vi "set shutdown.vi"(7 "system status in":T1={"system state"=enum."Empty & Closed", "fuel level"=0.0, "LOX level"=0.0, "system warnings"={"oxidizer overpress"=FALSE, "oxidizer leak"=FALSE, "fuel overpress"=FALSE, "fuel leak"=FALSE}, "valves"={"fuel load"=FALSE, "fuel return"=FALSE, "fuel comb"=FALSE, "fuel dump"=FALSE, "LOX load"=FALSE, "LOX return"=FALSE, "LOX comb"=FALSE, "LOX dump"=FALSE}, "ignition"=FALSE}) -> (8 "system status out":T1={"system state"=enum."Empty & Closed", "fuel level"=0.0, "LOX level"=0.0, "system warnings"={"oxidizer overpress"=FALSE, "oxidizer leak"=FALSE, "fuel overpress"=FALSE, "fuel leak"=FALSE}, "valves"={"fuel load"=FALSE, "fuel return"=FALSE, "fuel comb"=FALSE, "fuel dump"=FALSE, "LOX load"=FALSE, "LOX return"=FALSE, "LOX comb"=FALSE, "LOX dump"=FALSE}, "ignition"=FALSE})   [LabVIEW 2017]
doc: "This subVI handles the setup for the rocket engine simulation shut down state.\nIt sets the system warnings off, the ignition off, and the valves off.\n\nPaul K Dixon\nP350\nCSUSB"
uses:
  typedefs/sysyem status.ctl
  typedefs/system state.ctl
  typedefs/rocket system warnings.ctl
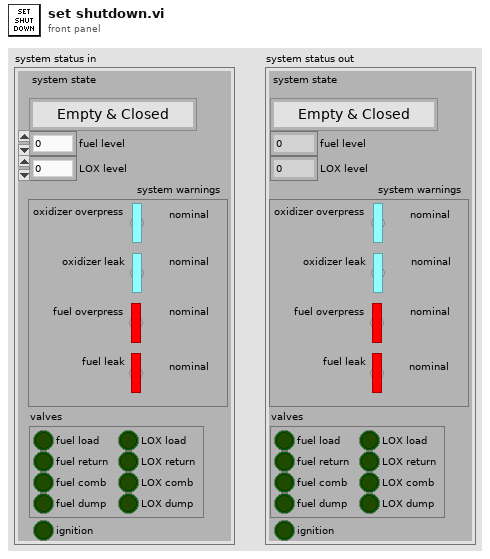
[diagram p1: front panel]
types:
  T1 = typedef "sysyem status.ctl" = cluster{"system state":T2, "fuel level":dbl, "LOX level":dbl, "system warnings":T3, "valves":cluster{"fuel load":bool, "fuel return":bool, "fuel comb":bool, "fuel dump":bool, "LOX load":bool, "LOX return":bool, "LOX comb":bool, "LOX dump":bool}, "ignition":bool}
  T2 = typedef "system state.ctl" = enum16{"Hold", "Empty & Closed", "Launch", "Return Fuel", "Return LOX", "Loading Lox", "Loading Fuel", "Shutdown", "Abort"}
  T3 = typedef "rocket system warnings.ctl" = cluster{"oxidizer overpress":bool, "oxidizer leak":bool, "fuel overpress":bool, "fuel leak":bool}
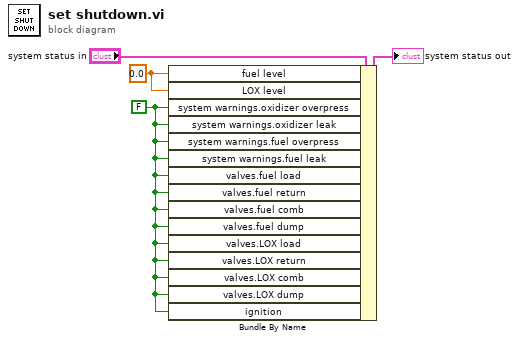
[diagram p0: block diagram]
diagram:
  w2 = 0.0 ("fuel level")
  w1 = FALSE ("system warnings.oxidizer overpress")
  n1 = Bundle By Name(cluster="system status in", "fuel level"=w2, "LOX level"=w2, "system warnings.oxidizer overpress"=w1, "system warnings.oxidizer leak"=w1, "system warnings.fuel overpress"=w1, "system warnings.fuel leak"=w1, "valves.fuel load"=w1, "valves.fuel return"=w1, "valves.fuel comb"=w1, "valves.fuel dump"=w1, "valves.LOX load"=w1, "valves.LOX return"=w1, "valves.LOX comb"=w1, "valves.LOX dump"=w1, "ignition"=w1) -> (→"system status out":T1)
